vi "eventHandler.vi"(8 "error in (no error)":errorcluster, 11 "Compiler in":refnum<class "Compiler.lvclass">) -> (0 "error out":errorcluster, 3 "Compiler out":refnum<class "Compiler.lvclass">)   [LabVIEW 2009, in "Compiler.lvlib" / "Compiler.lvclass"]
uses:
  Compiler.lvclass
  CompiledList/CompiledList.lvclass
  Compiler.lvclass/Compiler.ctl
  Hal/HWController/HWControllerEvents/HWControllerEvents.lvclass
panel:
  out "stop":bool
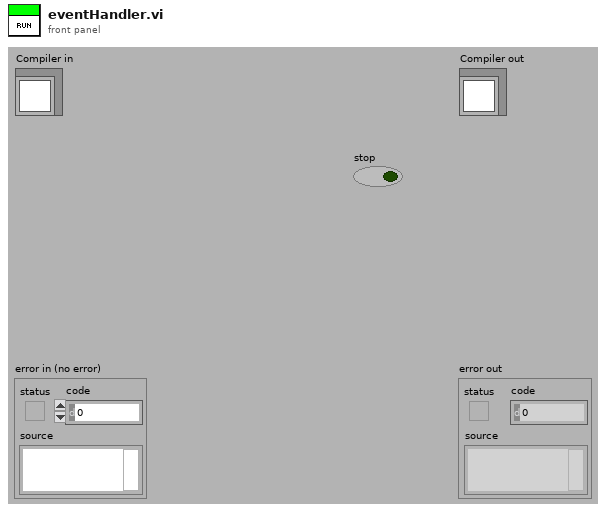
[diagram p1: front panel]
types:
  T1 = cluster{"Compiler in":refnum<class "Compiler.lvclass">, "Compiler.lvlib:CompiledList.lvclass":refnum<class "CompiledList.lvclass">}
  T2 = cluster{"incomingEventTypes":cluster{"start":cluster{"Boolean":bool}, "stop":cluster{"Boolean":bool}, "statusInquiry":cluster{"Boolean":bool}, "configure":cluster{"DPScriptPath":path, "TimeStamp":string, "HWLoop?":bool}, "resetError":cluster{"Boolean":bool}, "resourcesInquiry":cluster{"Boolean":bool}, "reserveResources":cluster{"HWList":string[]}, "initialise":cluster{"HWList":string[]}, "close":cluster{"Boolean":bool}, "resetAllChannels":cluster{"Boolean":bool}, "staticChannelUpdate":cluster{"channel_address":string, "calibratedValue":dbl}, "runScript":cluster{"DPScriptPath":path, "TimeStamp":string, "HWLoop?":bool}, "compilingScript":cluster{"Path":path}, "compiledScript":cluster{"Path":path, "timeCompileAt":string}, "compilerError":cluster{"Path":path}, "configureCompiledScript":cluster{"DPScriptPath":path, "TimeStamp":string, "HWLoop?":bool, "CompiledScript":cluster{"ScriptListCompiler.lvclass":refnum<class "ScriptListCompiler.lvclass">, "aoChannels":refnum<class "AnalogOutput.lvclass">[], "doChannels":refnum<class "DigitalOutput.lvclass">[], "rfChannels":refnum<class "DDSOutput.lvclass">[]}}, "restartCompiler":cluster{"restart":bool}, "staticRfChannelUpdate":cluster{"channel_address":string, "Output":cluster{"Frequency(MHz)":dbl, "Amplitude":dbl, "Phase":dbl, "OutputForm":enum16{"Sine", "Square", "Triangle", "Arbitrary"}}}, "cameraUpdate":cluster{"Camera":string, "Type":string, "settings":path}}, "outgoingEventTypes":cluster{"HWStatus":cluster{"status":enum16{"Ready", "Compiling", "Configured", "Running", "Stopping", "Unresolved Error"}}, "error":cluster{"error out":errorcluster}, "resourcesAvailable":cluster{"availableHWList":string[], "reservedHWList":string[]}, "resourcesReserved":cluster{"reservedHWList":string[]}}}
  T3 = enum16{"start", "stop", "statusInquiry", "configure", "resetError", "resourcesInquiry", "reserveResources", "initialise", "resetAllChannels", "staticUpdate", "close", "HWStatus", "error", "resourcesAvailable", "resourcesReserved", "compilerError", "compiledScript", "compilingScript", "runScript", "configureCompiledScript", "restartCompiler", "staticRfChannelUpdate", "cameraUpdate"}
  T4 = cluster{"Compiler out":refnum<class "Compiler.lvclass">, "CompiledList":refnum<class "CompiledList.lvclass">}
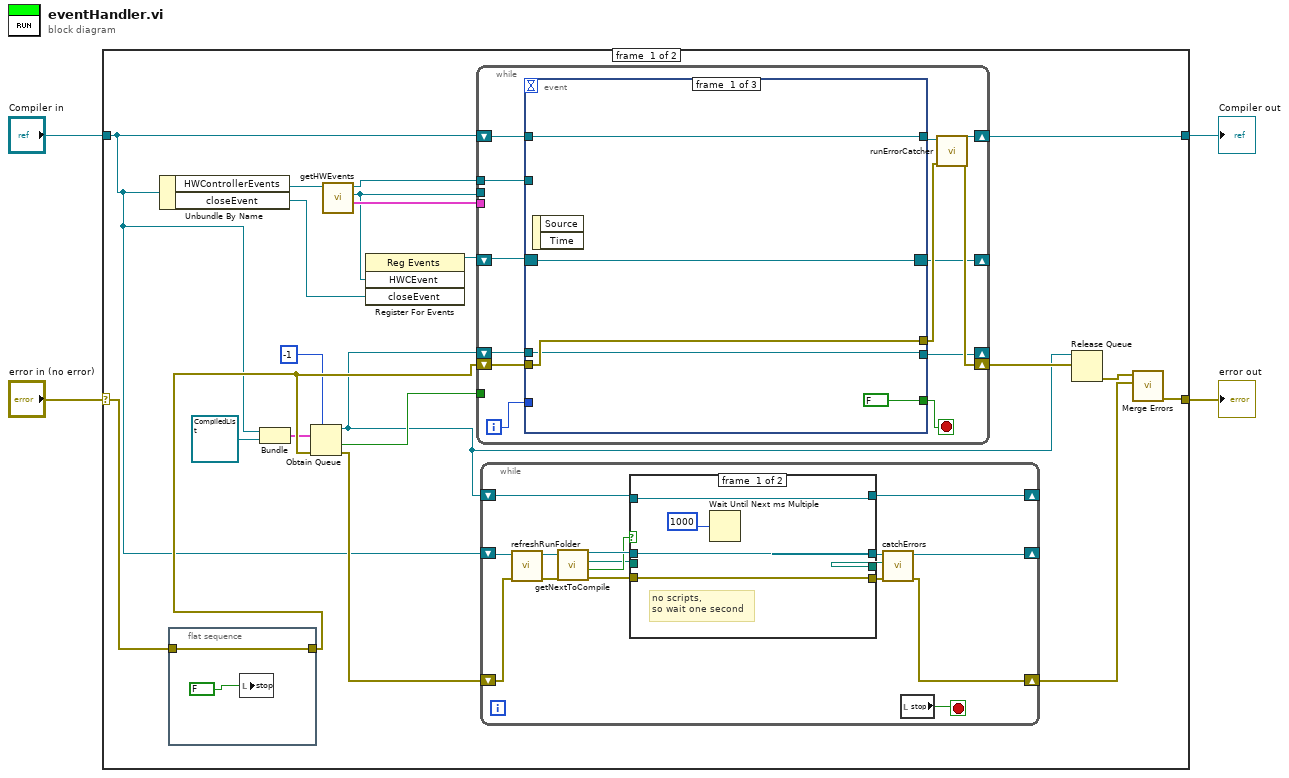
[diagram p0: block diagram]
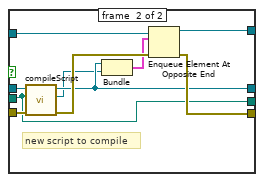
[diagram p2: hidden frame]
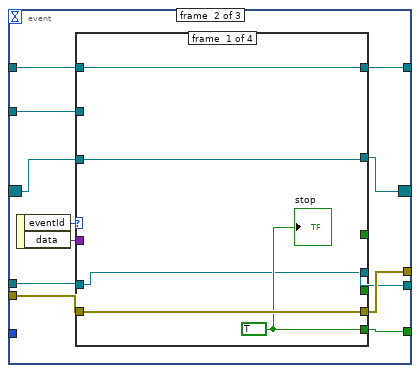
[diagram p3: hidden frame]
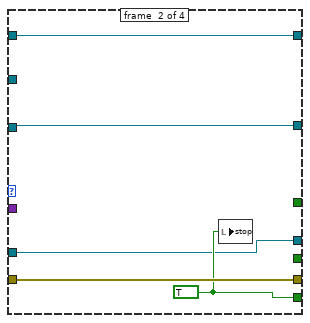
[diagram p4: hidden frame]
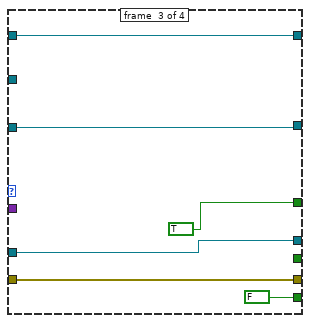
[diagram p5: hidden frame]
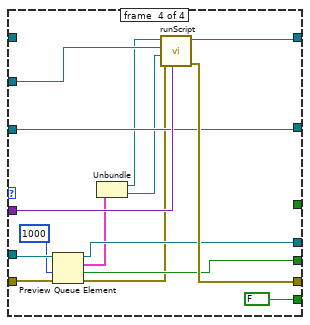
[diagram p6: hidden frame]
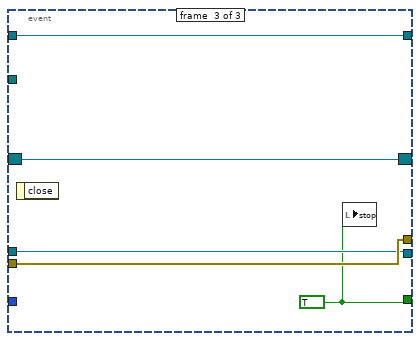
[diagram p7: hidden frame]
diagram:
  n1 = case shown="No Error" "error in (no error)" {
    selector: "error in (no error)" -> [w15 w124]
    tunnel: [w18 w124] -> w3
    tunnel: [w23 w123] -> w1
    tunnel: "Compiler in" -> [w6 w123]
    frame #0 {
      n2 = Unbundle By Name(w6) -> ("HWControllerEvents"=w24:refnum<class "HWControllerEvents.lvclass">, "closeEvent"=w5:refnum<user-event>)
      n3 = flat-sequence {
        tunnel: w15 -> [w25]
        tunnel: [w25] -> w14
        frame #0 {
          n4 = local write "stop"(FALSE) -> ()
        }
      }
      n5 = Bundle("Compiler in"=w6, "Compiler.lvlib:CompiledList.lvclass"=refnum<class "CompiledList.lvclass"> refnum) -> (w7:T1)  [unwired: 1 in]
      n6 = Obtain Queue(max queue size (-1, unlimited)=-1, element data type=w7, error in (no error)=w14) -> (queue out=w9:refnum<queue>, created new?=w10:bool, error out=w19:errorcluster)  [unwired: 2 in]
      n7 = call-dynamic "getHWEvents.vi"("HWControllerEvents in"=w24) -> ("eventDataTypes"=w21:T2, "HWCEvent"=w20:refnum<user-event>, "HWControllerEvents out"=w16:refnum<class "HWControllerEvents.lvclass">)  [unwired: 7 in, 1 out]
      n8 = register-events(w20, w5) -> (reference out=w22:refnum<event-registration>)  [unwired: 2 in, 1 out]
      n9 = while {
        shift-right: [w62] -> w23
        shift-left: w6 -> [w69]
        tunnel: w20 -> [_]
        tunnel: w21 -> [_]
        shift-right: [w60] -> w13
        shift-left: w14 -> [w67]
        tunnel: w16 -> [w64]
        shift-right: [w58] -> _
        shift-left: w22 -> [w68]
        tunnel: w10 -> [_]
        shift-right: [w57] -> _
        shift-left: w9 -> [w66]
        i -> [w59]
        stop <- w65 stop-if-true
        n10 = event shown="[2] <closeEvent>: User Event" {
          selector: w68 -> [w72 w78 w119]
          dyn-events: [w72 w77 w119] -> w58
          timeout: _ -> [_ _ _]
          tunnel: w69 -> [w74 w82 w120]
          tunnel: [w74 w83 w120] -> w63
          tunnel: w67 -> [w73 w85 w122]
          tunnel: [w73 w80 w122] -> w61
          tunnel: w66 -> [w70 w84 w121]
          tunnel: [FALSE w79 w118] -> w65
          tunnel: w64 -> [_ w81 _]
          tunnel: w59 -> [_ _ _]
          tunnel: [w70 w75 w121] -> w57
          event #0 {
            n11 = event-data() -> ()  [unwired: 1 in, 2 out]
          }
          event #1 {
            n12 = event-data() -> ("eventId"=w86:T3, "data"=w76:variant)  [unwired: 1 in]
            n13 = case shown="\"close\"" w86 {
              tunnel: w76 -> [_ _ _ w114]
              tunnel: w85 -> [w90 w96 w101 w110]
              tunnel: w84 -> [w87 w92 w97 w111]
              tunnel: [w91 w95 w102 w116] -> w83
              tunnel: w82 -> [w91 w95 w102 _]
              tunnel: w81 -> [_ _ _ w117]
              tunnel: [w90 w96 w101 w115] -> w80
              tunnel: [w89 w93 FALSE FALSE] -> w79
              tunnel: w78 -> [w88 w94 w100 w113]
              tunnel: [w88 w94 w100 w113] -> w77
              tunnel: [_ _ TRUE _] -> _
              tunnel: [_ _ _ w108] -> _
              tunnel: [w87 w92 w97 w107] -> w75
              frame #0 {
                w89 = TRUE
                "stop" <- w89
              }
              frame #1 {
                w93 = TRUE
                n14 = local write "stop"(w93) -> ()
              }
              frame #2 {
              }
              frame #3 {
                n15 = Preview Queue Element(queue=w111, timeout in ms (-1)=1000, error in (no error)=w110) -> (queue out=w107:refnum<queue>, element=w106:T1, timed out?=w108:bool, error out=w103:errorcluster)
                n16 = Unbundle(w106) -> ("Compiler in"=w105:refnum<class "Compiler.lvclass">, "Compiler.lvlib:CompiledList.lvclass"=w104:refnum<class "CompiledList.lvclass">)
                n17 = call "runScript.vi"("data"=w114, "error in (no error)"=w103, "CompiledList"=w104, "HWControllerEvents in"=w117, "Compiler in"=w105) -> ("error out"=w115:errorcluster, "Compiler out"=w116:refnum<class "Compiler.lvclass">)  [unwired: 5 in]
              }
            }
          }
          event #2 {
            w118 = TRUE
            n18 = event-data() -> ()  [unwired: 1 in, 1 out]
            n19 = local write "stop"(w118) -> ()
          }
        }
        n20 = call "runErrorCatcher.vi"("error in (no error)"=w61, "Compiler in"=w63) -> ("error out"=w60:errorcluster, "Compiler out"=w62:refnum<class "Compiler.lvclass">)  [unwired: 8 in]
      }
      n21 = while {
        shift-right: [w32] -> w17
        shift-left: w19 -> [w40]
        shift-right: [w29] -> _
        shift-left: w6 -> [w41]
        shift-right: [w27] -> _
        shift-left: w9 -> [w35]
        stop <- w42 stop-if-true
        n22 = call "refreshRunFolder.vi"("error in (no error)"=w40, "Compiler in"=w41) -> ("error out"=w38:errorcluster, "Compiler out"=w39:refnum<class "Compiler.lvclass">)  [unwired: 8 in]
        n23 = call "getNextToCompile.vi"("error in (no error)"=w38, "Compiler in"=w39) -> ("error out"=w37:errorcluster, "newScript?"=w31:bool, "Path"=w30:path, "Compiler out"=w36:refnum<class "Compiler.lvclass">)  [unwired: 6 in]
        n24 = case shown="True" w31 {
          tunnel: w37 -> [w45 w56]
          tunnel: w36 -> [w46 w55]
          tunnel: w35 -> [w43 w53]
          tunnel: [w46 w49] -> w34
          tunnel: [w45 w54] -> w33
          tunnel: w30 -> [_ w51]
          tunnel: [_ w51] -> w28
          tunnel: [w43 w50] -> w27
          frame #0 {
            # "no scripts,\nso wait one second"
            n25 = Wait Until Next ms Multiple(millisecond multiple=1000) -> ()  [unwired: 1 out]
          }
          frame #1 {
            # "new script to compile"
            n26 = call "compileScript.vi"("error in (no error)"=w56, "Path"=w51, "Compiler in"=w55) -> ("error out"=w52:errorcluster, "CompiledList"=w48:refnum<class "CompiledList.lvclass">, "Compiler out"=w49:refnum<class "Compiler.lvclass">)  [unwired: 6 in]
            n27 = Bundle("Compiler out"=w49, "CompiledList"=w48) -> (w47:T4)  [unwired: 1 in]
            n28 = Enqueue Element At Opposite End(queue=w53, element=w47, error in (no error)=w52) -> (queue out=w50:refnum<queue>, error out=w54:errorcluster)  [unwired: 1 in, 1 out]
          }
        }
        n29 = call "catchErrors.vi"("error in (no error)"=w33, "Path"=w28, "Compiler in"=w34) -> ("error out"=w32:errorcluster, "Compiler out"=w29:refnum<class "Compiler.lvclass">)  [unwired: 7 in]
        n30 = local read "stop"() -> (w42:bool)
      }
      n31 = Release Queue(queue=w9, error in (no error)=w13) -> (error out=w12:errorcluster)  [unwired: 1 in, 2 out]
      n32 = call <vilib>:"Merge Errors.vi"("error in 2 (no error)"=w17, "error in 1 (no error)"=w12) -> ("error out"=w18:errorcluster)  [unwired: 5 in]
    }
    frame #1 {
    }
  }
  "error out" <- w3
  "Compiler out" <- w1
